vi "CloseHardware.vi"(8 "error in (no error)":errorcluster, 11 "PCO in":refnum<class "PCO_Camera.lvclass">) -> (0 "error out":errorcluster, 3 "PCO out":refnum<class "PCO_Camera.lvclass">)   [LabVIEW 2020, in "PCO_Camera.lvclass"]
uses:
  PCO_Camera.lvclass
  PCO_Camera.lvclass/PCO_Camera.ctl
  Camera.lvclass
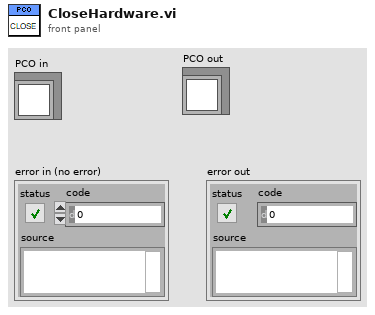
[diagram p1: front panel]
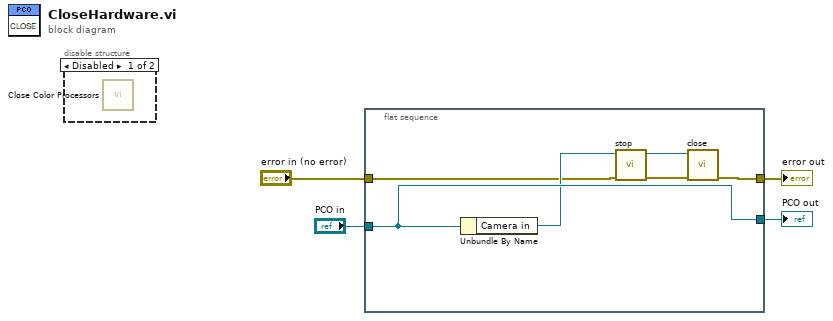
[diagram p0: block diagram]
diagram:
  n1 = disable-structure shown="Disabled" {
    frame Disabled {
      n2 = call "Close Color Processors.vi"() -> ()  [unwired: 11 in, 1 out]
    }
    frame Enabled {
    }
  }
  n3 = flat-sequence {
    tunnel: "PCO in" -> [w9]
    tunnel: "error in (no error)" -> [w7]
    tunnel: [w9] -> w2
    tunnel: [w10] -> w1
    frame #0 {
      n4 = Unbundle By Name(w9) -> ("Camera in"=w8:refnum<class "Camera.lvclass">)
      n5 = call-dynamic "stop.vi"("error in (no error)"=w7, "Camera in"=w8) -> ("error out"=w6:errorcluster, "Camera out"=w5:refnum<class "Camera.lvclass">)  [unwired: 8 in]
      n6 = call-dynamic "close.vi"("error in (no error)"=w6, "Camera in"=w5) -> ("error out"=w10:errorcluster)  [unwired: 9 in]
    }
  }
  "PCO out" <- w2
  "error out" <- w1
